vi "create_project_Dialog.vi"(10 "当前项目配置 输入":T1) -> (2 "当前项目配置 输出":T1)   [LabVIEW 2018, in "menu.lvlib"]
uses:
  menu.lvlib
panel:
  out "日期/时间字符串":string
  in  "项目名":string
  out "取消？":bool
  in  "取消按钮":bool
  in  "确定按钮":bool
  in  "项目文件路径":path
  in  "error in (no error)":cluster{"状态":bool, "代码":i32, "源":string} caption="错误输入（无错误）"
  out "error out":cluster{"状态":bool, "代码":i32, "源":string} caption="错误输出"
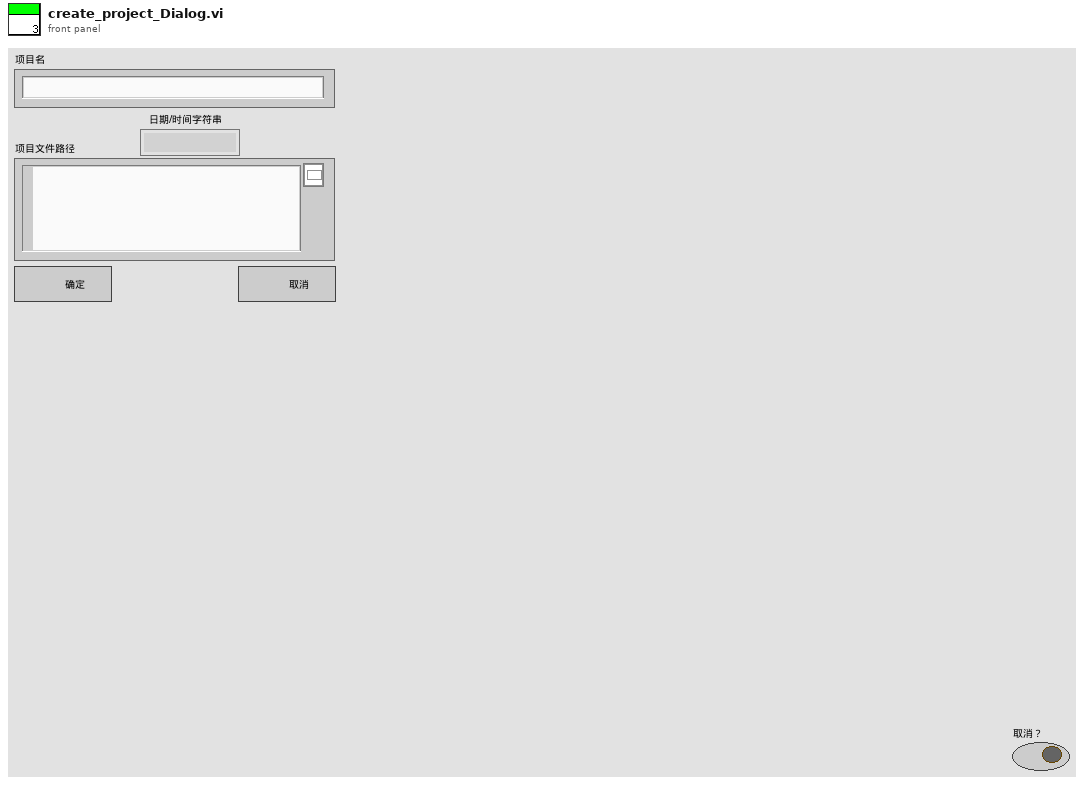
[diagram p1: front panel]
types:
  T1 = cluster{"控制参数配置":string, "模拟响应配置":string, "串口通信配置":string, "数据显示配置":string, "数据记录配置":string, "安全/报警配置":string, "模拟负载数据":string, "模拟加载数据":string, "总电源":bool, "电机1上电":bool, "电机2上电":bool, "串口连接":bool, "电机1\n相电流报警":bool, "电机2\n相电流报警":bool, "电机1\n母线电压报警":bool, "电机2\n母线电压报警":bool, "保存设置":bool, "从文件加载":bool, "恢复默认设置":bool, "路径":path, "项目路径":path, "项目名":string, "创建时间":string, "上次使用时间":string}
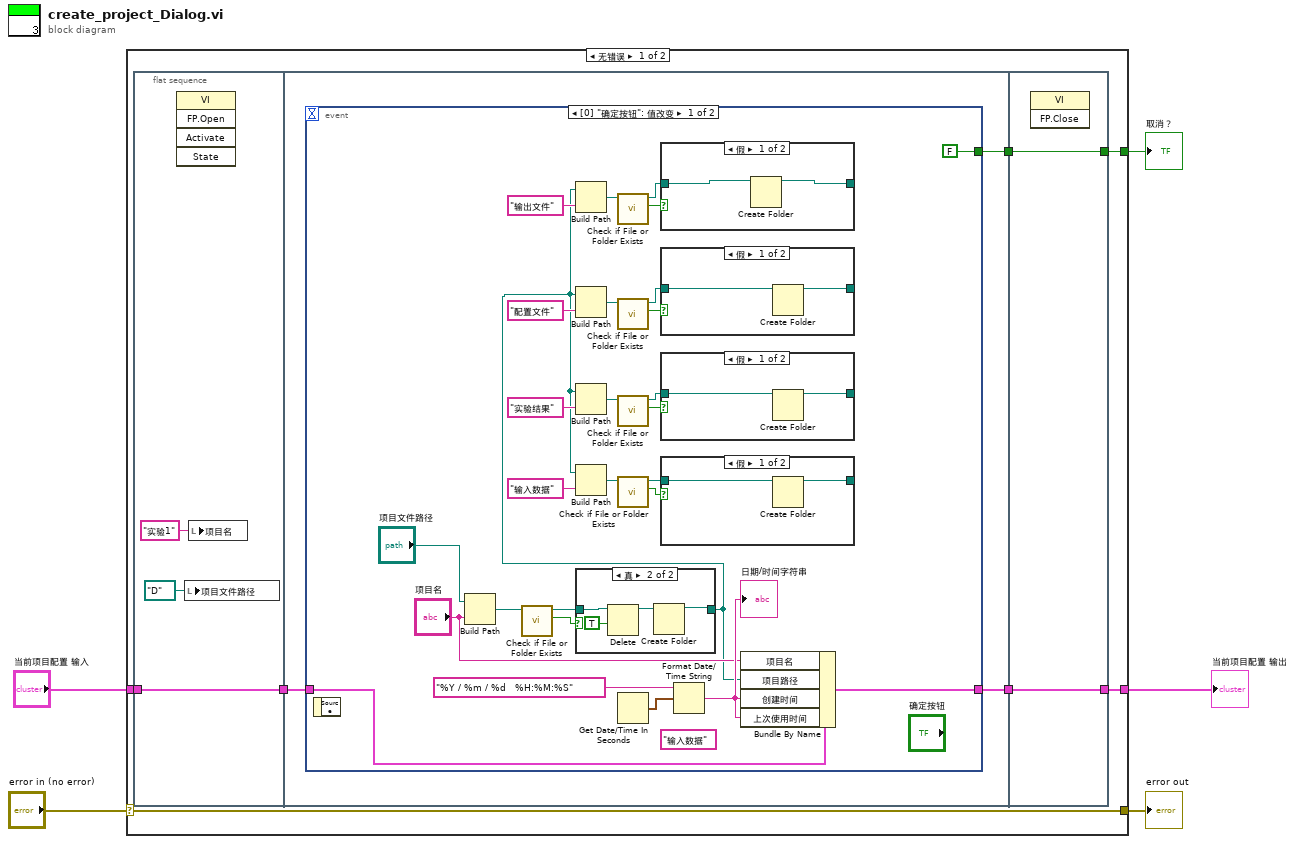
[diagram p0: block diagram]
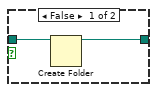
[diagram p6: hidden frame]
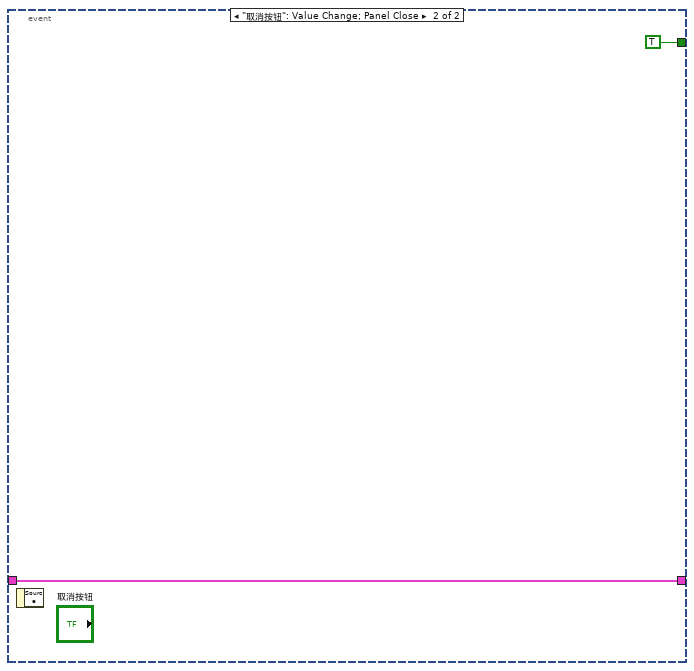
[diagram p7: hidden frame]
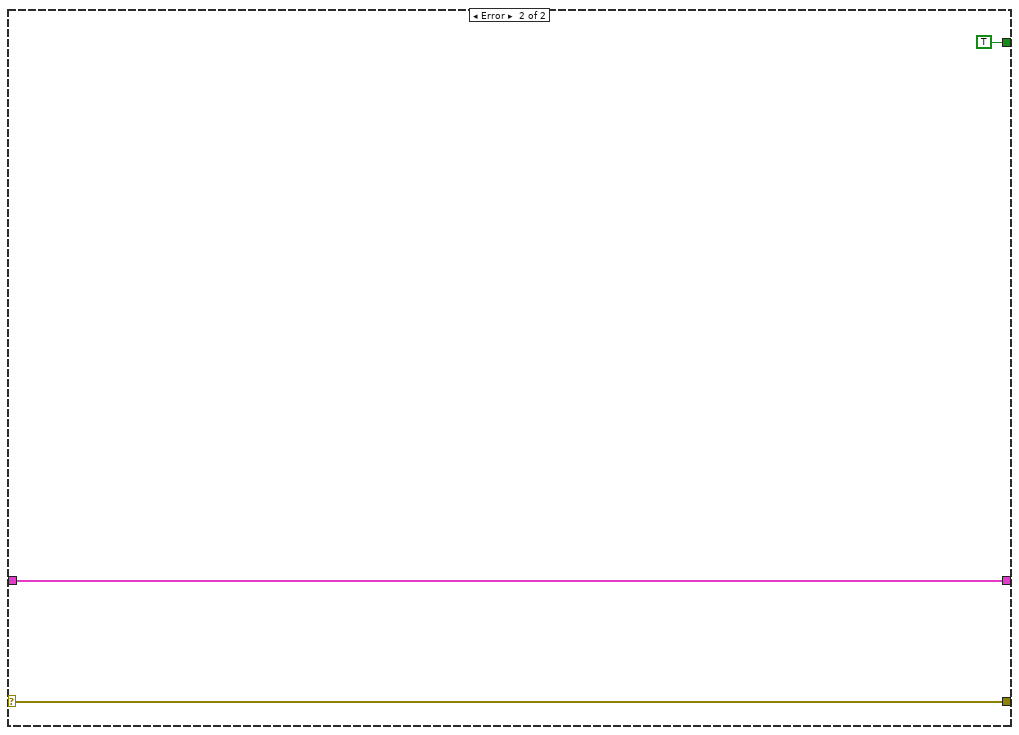
[diagram p8: hidden frame]
diagram:
  n1 = case shown="无错误" "error in (no error)" {
    selector: "error in (no error)" -> [w12 w71]
    tunnel: [w12 w71] -> w4
    tunnel: "当前项目配置 输入" -> [w6 w70]
    tunnel: [w10 w70] -> w1
    tunnel: [w11 TRUE ("UI Refresh Needed?")] -> w3
    frame No Error {
      n2 = flat-sequence {
        tunnel: w6 -> [w15]
        tunnel: [w15] -> w9
        tunnel: w9 -> [w16]
        tunnel: [w18] -> w8
        tunnel: [w17] -> w7
        tunnel: [w67] -> w10
        tunnel: [w68] -> w11
        tunnel: w8 -> [w68]
        tunnel: w7 -> [w67]
        frame #0 {
          n3 = invoke class="VI" method="FP.Open"() -> ()  [unwired: 5 in, 5 out]
          n4 = local write "项目文件路径"(path "D:/" ("项目文件路径")) -> ()
          n5 = local write "项目名"("实验1" ("项目名")) -> ()
        }
        frame #1 {
          n6 = event shown="[0] \"确定按钮\": 值改变" {
            selector: _ -> [_ _]
            dyn-events: _ -> [_ _]
            timeout: _ -> [_ _]
            tunnel: [w44 w66] -> w17
            tunnel: w16 -> [w45 w66]
            tunnel: [FALSE ("UI Refresh Needed?") TRUE ("UI Refresh Needed?")] -> w18
            event "确定按钮": Value Change {
              (unwired) "输入数据"
              n7 = event-data() -> ()  [unwired: 1 in, 1 out]
              n8 = Build Path(base path="项目文件路径", name or relative path="项目名") -> (appended path=w21:path)
              n9 = call <vilib>:"Check if File or Folder Exists.vi"("path"=w21) -> ("file or folder exists?"=w39:bool, "dup path"=w40:path)  [unwired: 8 in, 1 out]
              n10 = case shown="真" w39 {
                tunnel: w40 -> [w60 w64]
                tunnel: [w59 w61] -> w19
                frame False {
                  n11 = Create Folder(path (use dialog)=w60) -> (created path=w59:path)  [unwired: 2 in, 2 out]
                }
                frame True {
                  n12 = Delete(path (use dialog)=w64, entire hierarchy (F)=TRUE ("整个层次结构(F)")) -> (deleted path=w62:path)  [unwired: 3 in, 2 out]
                  n13 = Create Folder(path (use dialog)=w62) -> (created path=w61:path)  [unwired: 2 in, 2 out]
                }
              }
              n14 = Build Path(base path=w19, name or relative path="输出文件") -> (appended path=w31:path)
              n15 = Build Path(base path=w19, name or relative path="配置文件") -> (appended path=w34:path)
              n16 = Build Path(base path=w19, name or relative path="实验结果") -> (appended path=w28:path)
              n17 = Build Path(base path=w19, name or relative path="输入数据") -> (appended path=w24:path)
              n18 = call <vilib>:"Check if File or Folder Exists.vi"("path"=w31) -> ("file or folder exists?"=w32:bool, "dup path"=w33:path)  [unwired: 8 in, 1 out]
              n19 = call <vilib>:"Check if File or Folder Exists.vi"("path"=w34) -> ("file or folder exists?"=w35:bool, "dup path"=w36:path)  [unwired: 8 in, 1 out]
              n20 = call <vilib>:"Check if File or Folder Exists.vi"("path"=w28) -> ("file or folder exists?"=w29:bool, "dup path"=w30:path)  [unwired: 8 in, 1 out]
              n21 = call <vilib>:"Check if File or Folder Exists.vi"("path"=w24) -> ("file or folder exists?"=w25:bool, "dup path"=w26:path)  [unwired: 8 in, 1 out]
              n22 = Get Date/Time In Seconds() -> (seconds since 1Jan1904=w43:timestamp)
              n23 = case shown="假" w32 {
                tunnel: w33 -> [w54 w55]
                tunnel: [w53 w55] -> _
                frame False {
                  n24 = Create Folder(path (use dialog)=w54) -> (created path=w53:path)  [unwired: 2 in, 2 out]
                }
                frame True {
                }
              }
              n25 = case shown="假" w35 {
                tunnel: w36 -> [w57 w58]
                tunnel: [w56 w58] -> _
                frame False {
                  n26 = Create Folder(path (use dialog)=w57) -> (created path=w56:path)  [unwired: 2 in, 2 out]
                }
                frame True {
                }
              }
              n27 = case shown="假" w29 {
                tunnel: w30 -> [w51 w52]
                tunnel: [w50 w52] -> _
                frame False {
                  n28 = Create Folder(path (use dialog)=w51) -> (created path=w50:path)  [unwired: 2 in, 2 out]
                }
                frame True {
                }
              }
              n29 = case shown="假" w25 {
                tunnel: w26 -> [w48 w49]
                tunnel: [w47 w49] -> _
                frame False {
                  n30 = Create Folder(path (use dialog)=w48) -> (created path=w47:path)  [unwired: 2 in, 2 out]
                }
                frame True {
                }
              }
              n31 = Format Date/Time String(time format string (%c)="%Y / %m / %d   %H:%M:%S" ("时间格式字符串(%c)"), seconds (now)=w43) -> (date/time string=w41:string)  [unwired: 1 in]
              "日期/时间字符串" <- w41
              n32 = Bundle By Name(cluster=w45, "项目名"="项目名", "项目路径"=w19, "创建时间"=w41, "上次使用时间"=w41) -> (w44:T1)
            }
            event "取消按钮": Value Change; Panel Close {
              n33 = event-data() -> ()  [unwired: 1 in, 1 out]
            }
          }
        }
        frame #2 {
          n34 = invoke class="VI" method="FP.Close"() -> ()  [unwired: 3 in, 3 out]
        }
      }
    }
    frame Error {
    }
  }
  "error out" <- w4
  "取消？" <- w3
  "当前项目配置 输出" <- w1
